vi "API.vi"(8 "error in (no error)":errorcluster, 11 "API Provider in":refnum<class "API Provider.lvclass">) -> (0 "error out":errorcluster, 2 "API":refnum<class "API.lvclass">, 3 "API Provider out":refnum<class "API Provider.lvclass">)   [LabVIEW 2020, in "Volatus.lvlib" / "API Provider.lvclass"]
uses:
  API Provider.lvclass
  API/API.lvclass
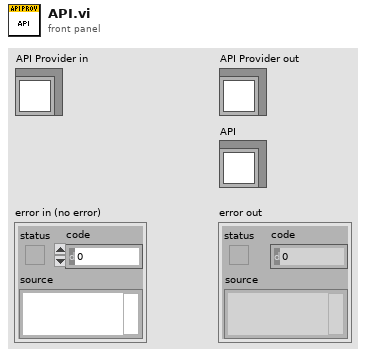
[diagram p1: front panel]
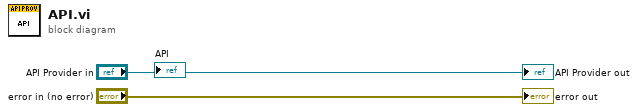
[diagram p0: block diagram]
diagram:
  "error out" <- "error in (no error)"
  "API Provider out" <- "API Provider in"
